vi "Wait for Command.vi"(6 "Synchronication":enum16{"Start", "Wait"}(ring), 8 "Command Info in":T1, 9 "Allocated":bool) -> (0 "Command Info out":T1)   [LabVIEW 2025]
doc: "If this command is supposed to wait until the controller to completes the operation, then wait for the Notifier, other return before it is complete."
uses:
  <vilib>/Rock Robotics/WPI/Framework/Command Status Info.ctl
  <vilib>/Rock Robotics/WPI/Framework/Completion Status.ctl
  <vilib>/Rock Robotics/WPI/Framework/Completion Notifier.ctl
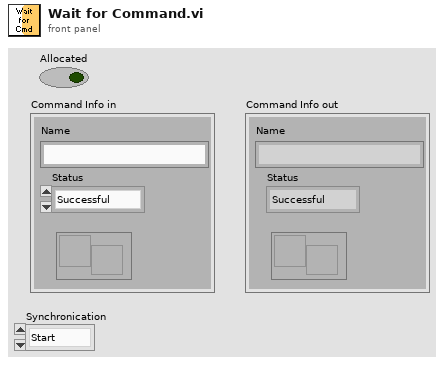
[diagram p1: front panel]
types:
  T1 = typedef "Command Status Info.ctl" = cluster{"Name":string, "Status":T2, "notifier out":T3}
  T2 = typedef "Completion Status.ctl" = enum16{"Successful", "Aborted", "Incomplete"}
  T3 = typedef "Completion Notifier.ctl" = refnum<notifier>
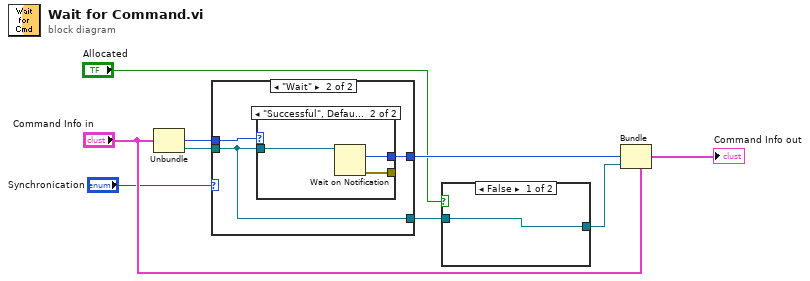
[diagram p0: block diagram]
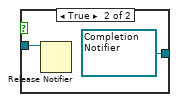
[diagram p2: hidden frame]
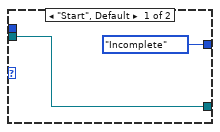
[diagram p3: hidden frame]
diagram:
  n1 = Unbundle("Command Info in") -> ("Status"=w1:T2, "notifier out"=w9:T3)  [unwired: 1 out]
  n2 = case shown="\"Wait\"" "Synchronication" {
    tunnel: w9 -> [w10 w13]
    tunnel: [Completion_Status."Incomplete" ("Completion Status") w14] -> w7
    tunnel: [w10 w13] -> w3
    tunnel: w1 -> [_ w12]
    frame "Start", Default {
    }
    frame "Wait" {
      n3 = case shown="\"Successful\", Default" w12 {
        selector: w12 -> [w15 _]
        tunnel: [w15 w18] -> w14
        tunnel: w13 -> [_ w17]
        tunnel: [_ w16] -> _
        frame "Aborted" {
        }
        frame "Successful", Default {
          n4 = Wait on Notification(notifier=w17) -> (notification=w18:T2, error out=w16:errorcluster)  [unwired: 3 in, 2 out]
        }
      }
    }
  }
  n5 = case shown="False" "Allocated" {
    tunnel: [w19 w21] -> w4
    tunnel: w3 -> [w19 w20]
    frame False {
    }
    frame True {
      w21 = T3 refnum items=["Successful", "Aborted", "Incomplete"] ("notifier out")
      n6 = Release Notifier(notifier=w20) -> ()  [unwired: 2 in, 3 out]
    }
  }
  n7 = Bundle(cluster="Command Info in", "Status"=w7, "notifier out"=w4) -> (→"Command Info out":T1)  [unwired: 1 in]
